vi "RPC Server-RT.vi"() -> ()   [LabVIEW 2020]
uses:
  <vilib>/Utility/error.llb/DialogType.ctl
  Lib/JSON-RPC/Classes/Server/Send Request (Sync).vi
  <vilib>/addons/analyzer/_analyzerutils.llb/VIAnUtil Check Type If ErrClust.vi
  Lib/JSON-RPC/Classes/Server/Add Response (Result).vi
  Lib/JSON-RPC/Classes/Server/Add Response (Internal Error).vi
  Lib/JSON-RPC/Classes/Server/Add Response (Method Not Found).vi
  Lib/JSON-RPC/Classes/Server/Add Response (Result from Request).vi
  Lib/JSON-RPC/Classes/Server/Add Response (Method Not Found from Request).vi
  Lib/JSON-RPC/Classes/Server/Add Response (Server Error from Request).vi
  Lib/JSON-RPC/Classes/Server/Add Response (Internal Error from Request).vi
  Lib/JSON-RPC/Classes/Server/JSONRPC Server.lvclass
  Controller/Controller.lvclass
  <vilib>/Utility/Data Type/NI_Data Type.lvlib
  <vilib>/NI_Real-Time Target Support.lvlib
  <vilib>/nisyscfg/nisyscfg.lvlib
panel:
  out "IP address":string
  out "header":string
  out "request":string
  out "response":string
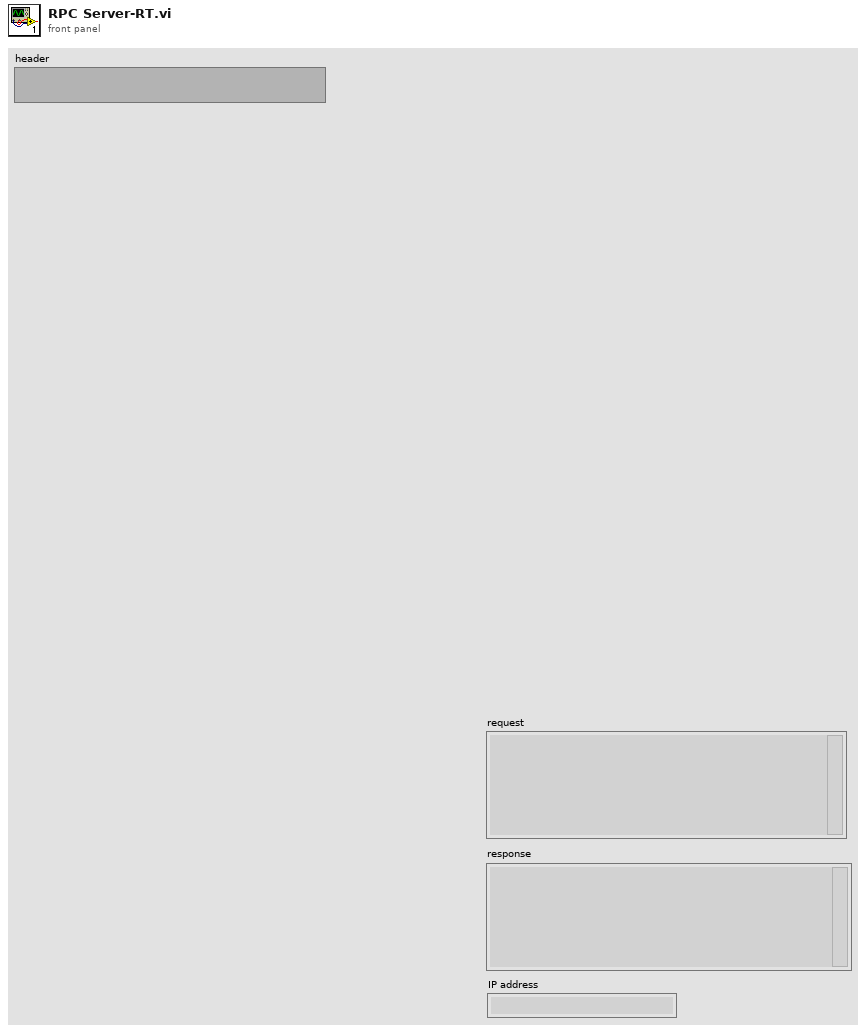
[diagram p1: front panel]
types:
  T1 = enum16{"Standard", "Buffered", "CRLF", "Immediate"}
  T2 = typedef "DialogType.ctl" = u16
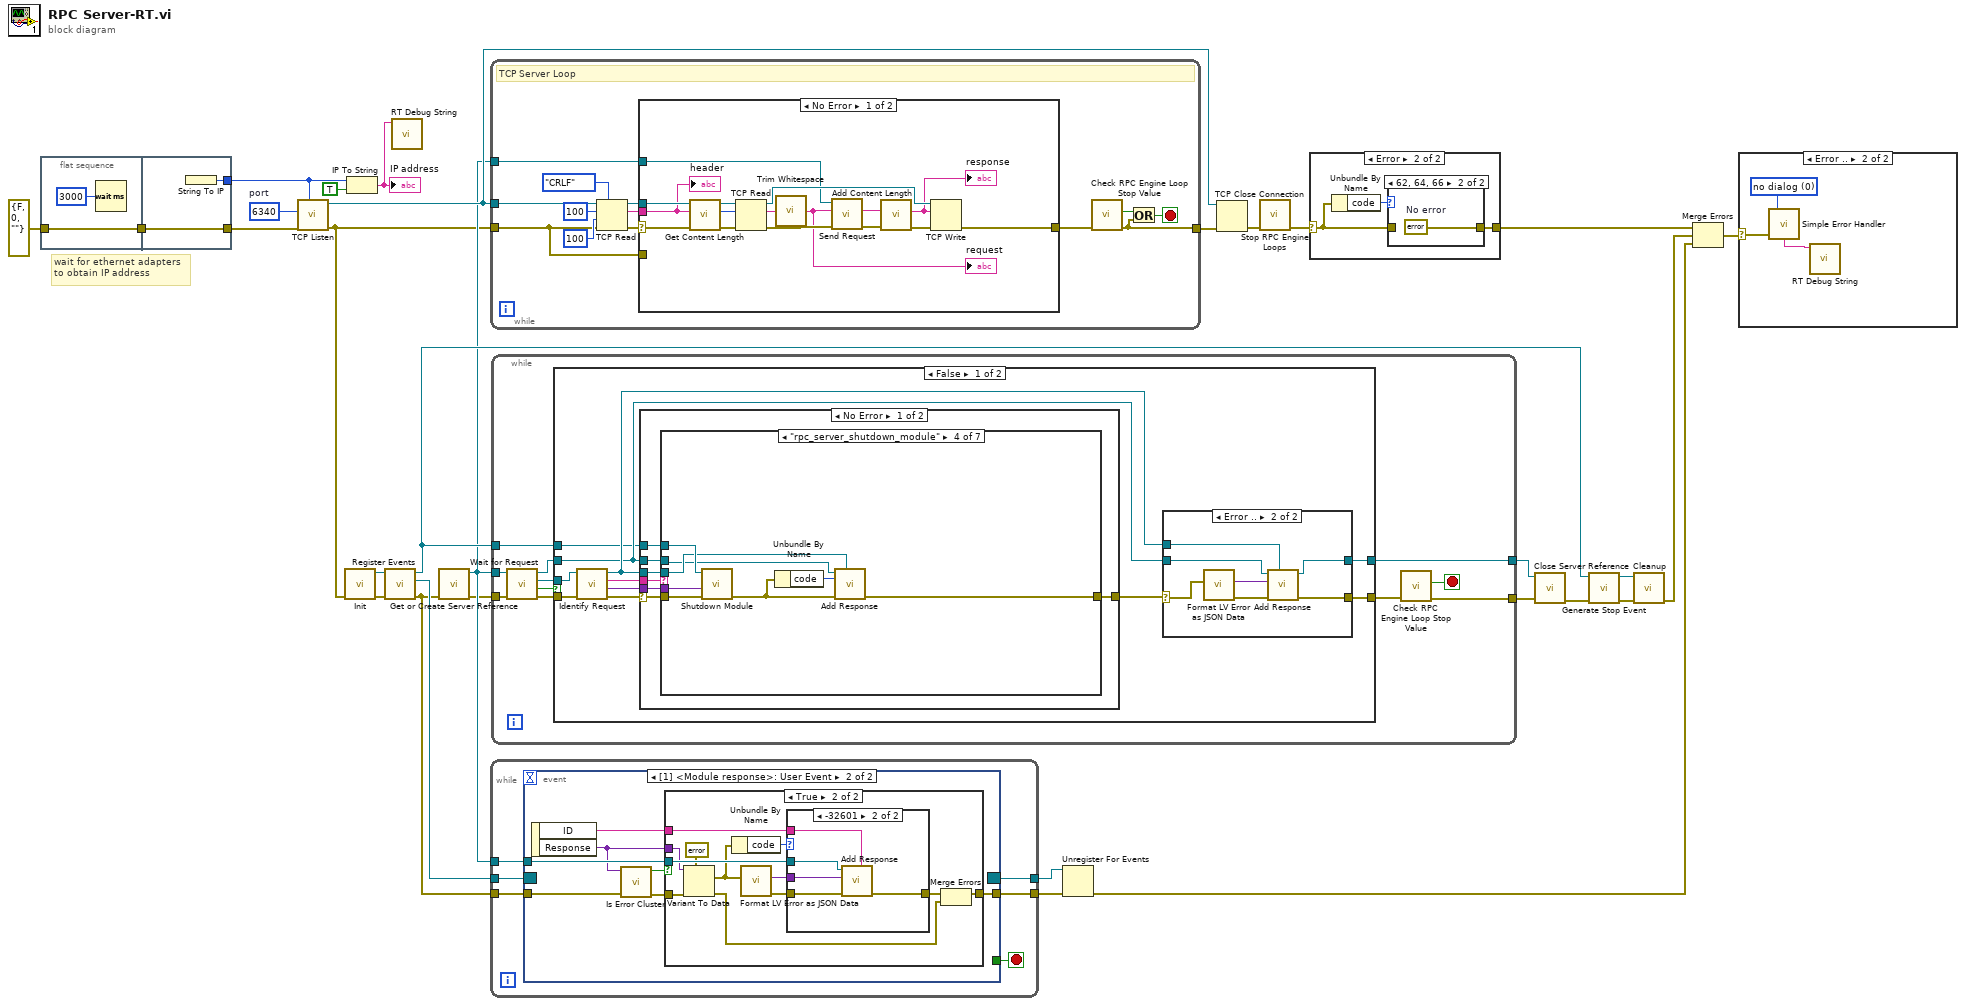
[diagram p0: block diagram]
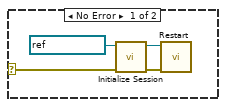
[diagram p2: hidden frame]
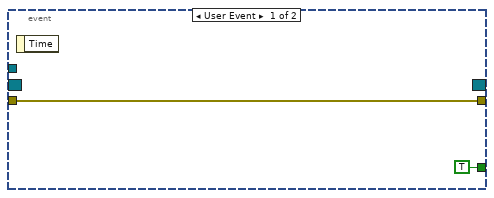
[diagram p3: hidden frame]
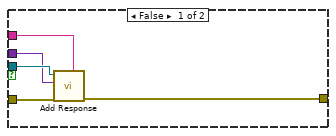
[diagram p4: hidden frame]
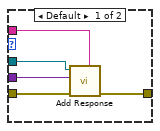
[diagram p5: hidden frame]
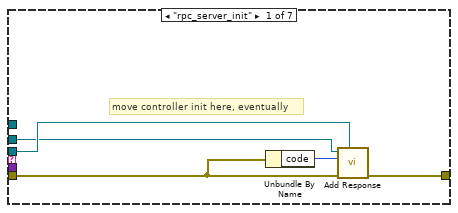
[diagram p7: hidden frame]
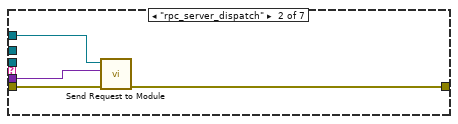
[diagram p8: hidden frame]
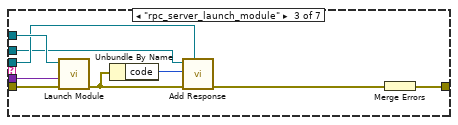
[diagram p9: hidden frame]
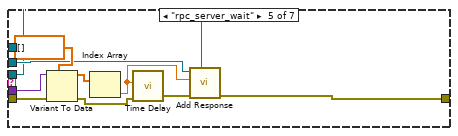
[diagram p10: hidden frame]
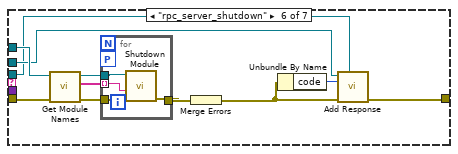
[diagram p11: hidden frame]
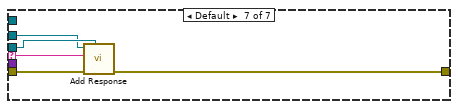
[diagram p12: hidden frame]
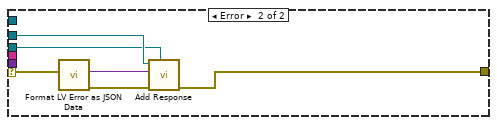
[diagram p13: hidden frame]
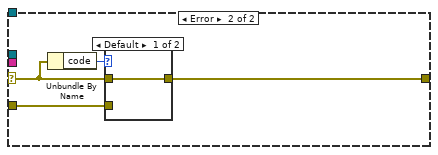
[diagram p17: hidden frame]
diagram:
  w29 = u16 6340  # port
  # "wait for ethernet adapters\nto obtain IP address"
  n1 = flat-sequence {
    tunnel: errorcluster {"status"=FALSE, "code"=0, "source"=""} ("error in (no error)") -> [w32]
    tunnel: [w32] -> w3
    tunnel: [w34] -> w6
    tunnel: w3 -> [w34]
    tunnel: [w33] -> w2
    frame #0 {
      n2 = Wait (ms)(milliseconds to wait=u32 3000) -> ()  [unwired: 1 out]
    }
    frame #1 {
      n3 = String To IP() -> (0:w33:u32)  [unwired: 1 in]
    }
  }
  n4 = call <vilib>:"TCP Listen.vi"("net address"=w2, "error in (no error)"=w6, "port"=w29) -> ("error out"=w4:errorcluster, "connection ID"=w26:refnum<k5>)  [unwired: 4 in, 3 out]
  n5 = call "Init.vi"("error in (no error)"=w4) -> ("error out"=w24:errorcluster, "Controller out"=w23:refnum<class "Controller.lvclass">)  [unwired: 9 in]
  n6 = IP To String(1:TRUE ("dot notation? (F)"), 2:w2) -> (0:w5:string)
  "IP address" <- w5
  n7 = call "Register Events.vi"("error in (no error)"=w24, "Controller in"=w23) -> ("error out"=w10:errorcluster, "Event Registration Refnum"=w22:refnum<event-registration>, "Controller out"=w15:refnum<class "Controller.lvclass">)  [unwired: 7 in]
  n8 = call <vilib>:"RT Debug String.vi"("String to write"=w5) -> ()  [unwired: 10 in, 1 out]
  n9 = call "Get or Create Server Reference.vi"("error in (no error)"=w10) -> ("error out"=w9:errorcluster, "Server Out"=w14:refnum<class "JSONRPC Server.lvclass">)  [unwired: 9 in]
  n10 = while {
    tunnel: [w35] -> w30
    tunnel: w26 -> [w41]
    tunnel: w4 -> [w42]
    tunnel: w14 -> [w39]
    stop <- w38 stop-if-true
    # "TCP Server Loop"
    n11 = TCP Read(connection ID=w41, bytes to read=100, error in (no error)=w42, 7:T1."CRLF" ("mode (standard)"), 9:100 ("timeout ms (25000)")) -> (connection ID out=w45:refnum<k5>, data out=w40:string, error out=w44:errorcluster)
    n12 = case shown="No Error" w44 {
      selector: w44 -> [w62 w65]
      tunnel: [w57 w64] -> w37
      tunnel: w42 -> [_ w63]
      tunnel: w45 -> [w60 _]
      tunnel: w40 -> [w59 _]
      tunnel: w39 -> [w51 _]
      frame No Error {
        n13 = call "Get Content Length.vi"("error in (no error)"=w62, "header"=w59) -> ("error out"=w61:errorcluster, "content length"=w58:i32)  [unwired: 8 in]
        n14 = TCP Read(connection ID=w60, bytes to read=w58, error in (no error)=w61) -> (connection ID out=w56:refnum<k5>, data out=w53:string, error out=w52:errorcluster)  [unwired: 2 out]
        n15 = call <vilib>:"Trim Whitespace.vi"("string"=w53) -> ("trimmed string"=w50:string)  [unwired: 1 in]
        "request" <- w50
        n16 = call-poly "Send Request.vi"("error in (no error)"=w52, "JSON Request String"=w50, "JSONRPC Server in"=w51) -> ("error out"=w48:errorcluster, "JSON Response String"=w49:string)  [unwired: 6 in, 1 out]
        n17 = call "Add Content Length.vi"("error in (no error)"=w48, "JSON Response String in"=w49) -> ("error out"=w55:errorcluster, "JSON Response String out"=w54:string)  [unwired: 8 in]
        "response" <- w54
        n18 = TCP Write(connection ID=w56, data in=w54, error in (no error)=w55) -> (error out=w57:errorcluster)  [unwired: 1 in, 2 out]
        "header" <- w59
      }
      frame Error {
        n19 = Unbundle By Name(w65) -> ("code"=w66:i32)
        n20 = case shown="Default" w66 {
          tunnel: w65 -> [w67 _]
          tunnel: w63 -> [_ w68]
          tunnel: [w67 w68] -> w64
          frame Default {
          }
          frame 56 {
          }
        }
      }
    }
    n21 = call "Check RPC Engine Loop Stop Value.vi"("error in (no error)"=w37) -> ("error out"=w35:errorcluster, "stopped?"=w36:bool)  [unwired: 9 in]
    n22 = Or(x=w36, y=w35) -> (x .or. y?=w38:bool)
  }
  n23 = while {
    tunnel: w22 -> [w74]
    tunnel: [w73] -> w21
    tunnel: w14 -> [w72]
    tunnel: w10 -> [w71]
    tunnel: [w70] -> w19
    stop <- w69 stop-if-true
    n24 = event shown="[1] <Module response>: User Event" {
      selector: w74 -> [_ _]
      dyn-events: [_ _] -> w73
      timeout: _ -> [_ _]
      tunnel: w72 -> [_ w81]
      tunnel: w71 -> [w76 w80]
      tunnel: [w76 w83] -> w70
      tunnel: [TRUE _] -> w69
      event User Event {
        n25 = event-data() -> ()  [unwired: 1 in, 1 out]
      }
      event User Event {
        n26 = event-data() -> ("ID"=w82:string, "Response"=w78:variant)  [unwired: 1 in]
        n27 = call <vilib>:"Is Error Cluster.vi"("error in (no error)"=w80, "variant"=w78) -> ("error out"=w79:errorcluster, "is error cluster?"=w77:bool)  [unwired: 8 in]
        n28 = case shown="True" w77 {
          tunnel: [w88 w98] -> w83
          tunnel: w82 -> [w87 w100]
          tunnel: w81 -> [w86 w99]
          tunnel: w79 -> [w85 w96]
          tunnel: w78 -> [w84 w94]
          frame False {
            n29 = call-poly "Add Response.vi"("id value"=w87, "error in (no error)"=w85, "JSON Value in"=w84, "Server in"=w86) -> ("error out"=w88:errorcluster)  [unwired: 5 in, 2 out]
          }
          frame True {
            n30 = Variant To Data(error in=w96, type=errorcluster {"status"=FALSE, "code"=0, "source"=""} ("data"), Variant=w94) -> (data=w91:errorcluster, error out=w95:errorcluster)
            n31 = Unbundle By Name(w91) -> ("code"=w92:i32)
            n32 = call "Format LV Error as JSON Data.vi"("error in"=w91) -> ("error out"=w89:errorcluster, "Error Value out"=w90:variant)  [unwired: 9 in]
            n33 = case shown="-32601" w92 {
              tunnel: w100 -> [w103 w108]
              tunnel: w99 -> [w105 w110]
              tunnel: [w104 w109] -> w97
              tunnel: w90 -> [w102 w107]
              tunnel: w89 -> [w101 w106]
              frame Default {
                n34 = call-poly "Add Response.vi"("id value"=w103, "error in (no error)"=w101, "JSON Value in"=w102, "Server in"=w105) -> ("error out"=w104:errorcluster)  [unwired: 5 in, 2 out]
              }
              frame -32601 {
                n35 = call-poly "Add Response.vi"("id value"=w108, "error in (no error)"=w106, "data"=w107, "Server in"=w110) -> ("error out"=w109:errorcluster)  [unwired: 5 in, 2 out]
              }
            }
            n36 = Merge Errors(w97, w95) -> (w98:errorcluster)
          }
        }
      }
    }
  }
  n37 = while {
    tunnel: w9 -> [w121]
    tunnel: w14 -> [w120]
    tunnel: [w112] -> w28
    tunnel: [w115] -> w27
    tunnel: w15 -> [w113]
    stop <- w111 stop-if-true
    n38 = call "Wait for Request.vi"("error in (no error)"=w121, "Server in"=w120) -> ("error out"=w119:errorcluster, "timed out?"=w116:bool, "Request"=w118:refnum<class "Request.lvclass">, "Server out"=w117:refnum<class "JSONRPC Server.lvclass">)  [unwired: 6 in]
    n39 = case shown="False" w116 {
      tunnel: w119 -> [w125 w212]
      tunnel: w118 -> [w132 _]
      tunnel: w117 -> [w123 w211]
      tunnel: [w128 w212] -> w114
      tunnel: [w127 w211] -> w115
      tunnel: w113 -> [w122 _]
      frame False {
        n40 = call "Identify Request.vi"("error in (no error)"=w125, "Request in"=w132) -> ("error out"=w126:errorcluster, "params"=w131:variant, "method"=w124:string, "Request out"=w129:refnum<class "Request.lvclass">)  [unwired: 5 in, 1 out]
        n41 = case shown="No Error" w126 {
          selector: w126 -> [w146 w210]
          tunnel: w131 -> [w143 _]
          tunnel: w123 -> [w148 w208]
          tunnel: w129 -> [w147 w207]
          tunnel: [w145 w205] -> w130
          tunnel: w124 -> [w144 _]
          tunnel: w122 -> [w142 _]
          frame No Error {
            n42 = case shown="\"rpc_server_shutdown_module\"" w144 {
              selector: w144 -> [_ _ _ _ _ _ w201]
              tunnel: w148 -> [w151 _ w160 w167 w178 w187 w202]
              tunnel: w147 -> [w152 _ w161 w168 w176 w185 w204]
              tunnel: w146 -> [w150 w157 w166 w174 w184 w190 w203]
              tunnel: [w153 w155 w165 w169 w175 w186 w200] -> w145
              tunnel: w143 -> [_ w154 w163 w172 w183 _ _]
              tunnel: w142 -> [_ w156 w164 w173 _ w191 _]
              frame "rpc_server_init" {
                # "move controller init here, eventually"
                n43 = Unbundle By Name(w150) -> ("code"=w149:i32)
                n44 = call-poly "Add Response.vi"("Request"=w152, "error in (no error)"=w150, "JSON Value in"=w149, "Server in"=w151) -> ("error out"=w153:errorcluster)  [unwired: 5 in, 2 out]
              }
              frame "rpc_server_dispatch" {
                n45 = call "Send Request to Module.vi"("error in (no error)"=w157, "Request"=w154, "Controller in"=w156) -> ("error out"=w155:errorcluster)  [unwired: 6 in, 2 out]
              }
              frame "rpc_server_launch_module" {
                n46 = call "Launch Module.vi"("error in (no error)"=w166, "params"=w163, "Controller in"=w164) -> ("error out"=w159:errorcluster)  [unwired: 7 in, 1 out]
                n47 = Unbundle By Name(w159) -> ("code"=w158:i32)
                n48 = call-poly "Add Response.vi"("Request"=w161, "error in (no error)"=w159, "JSON Value in"=w158, "Server in"=w160) -> ("error out"=w162:errorcluster)  [unwired: 5 in, 2 out]
                n49 = Merge Errors(w162) -> (w165:errorcluster)
              }
              frame "rpc_server_shutdown_module" {
                n50 = call "Shutdown Module.vi"("error in (no error)"=w174, "params"=w172, "Controller in"=w173) -> ("error out"=w170:errorcluster)  [unwired: 7 in, 1 out]
                n51 = Unbundle By Name(w170) -> ("code"=w171:i32)
                n52 = call-poly "Add Response.vi"("Request"=w168, "error in (no error)"=w170, "JSON Value in"=w171, "Server in"=w167) -> ("error out"=w169:errorcluster)  [unwired: 5 in, 2 out]
              }
              frame "rpc_server_wait" {
                n53 = Variant To Data(error in=w184, type=dbl[] [], Variant=w183) -> (data=w181:dbl[], error out=w180:errorcluster)
                n54 = Index Array(array=w181) -> (element=w177:dbl)  [unwired: 1 in]
                n55 = call "Time Delay"("error in (no error)"=w180, "Delay Time (s)"=w177) -> ("error out"=w179:errorcluster)  [unwired: 9 in]
                n56 = call-poly "Add Response.vi"("Request"=w176, "error in (no error)"=w179, "JSON Value in"=w177, "Server in"=w178) -> ("error out"=w175:errorcluster)  [unwired: 5 in, 2 out]
              }
              frame "rpc_server_shutdown" {
                n57 = call "Get Module Names.vi"("error in (no error)"=w190, "Controller in"=w191) -> ("error out"=w194:errorcluster, "Names"=w195:string[], "Controller out"=w192:refnum<class "Controller.lvclass">)  [unwired: 7 in]
                n58 = for {
                  tunnel: w192 -> [w199]
                  tunnel: w195 -> [w196] mode=indexing
                  tunnel: w194 -> [w198]
                  tunnel: [w197] -> _ mode=indexing
                  tunnel: [w197] -> w193
                  workers-P: _ -> [_]
                  n59 = call "Shutdown Module.vi"("error in (no error)"=w198, "params"=w196, "Controller in"=w199) -> ("error out"=w197:errorcluster)  [unwired: 7 in, 1 out]
                }
                n60 = Merge Errors(w193) -> (w189:errorcluster)
                n61 = Unbundle By Name(w189) -> ("code"=w188:i32)
                n62 = call-poly "Add Response.vi"("Request"=w185, "error in (no error)"=w189, "JSON Value in"=w188, "Server in"=w187) -> ("error out"=w186:errorcluster)  [unwired: 5 in, 2 out]
              }
              frame Default {
                n63 = call-poly "Add Response.vi"("Request"=w204, "error in (no error)"=w203, "data"=w201, "Server in"=w202) -> ("error out"=w200:errorcluster)  [unwired: 5 in, 2 out]
              }
            }
          }
          frame Error {
            n64 = call "Format LV Error as JSON Data.vi"("error in"=w210) -> ("error out"=w209:errorcluster, "Error Value out"=w206:variant)  [unwired: 9 in]
            n65 = call-poly "Add Response.vi"("Request"=w207, "error in (no error)"=w209, "data"=w206, "Server in"=w208) -> ("error out"=w205:errorcluster)  [unwired: 5 in, 2 out]
          }
        }
        n66 = case shown="Error .." w130 {
          selector: w130 -> [w134 w139]
          tunnel: [w134 w138] -> w128
          tunnel: w123 -> [w133 w136]
          tunnel: [w133 w137] -> w127
          tunnel: w129 -> [_ w135]
          frame No Error {
          }
          frame Error {
            n67 = call "Format LV Error as JSON Data.vi"("error in"=w139) -> ("error out"=w141:errorcluster, "Error Value out"=w140:variant)  [unwired: 9 in]
            n68 = call-poly "Add Response.vi"("Request"=w135, "error in (no error)"=w141, "data"=w140, "Server in"=w136) -> ("error out"=w138:errorcluster, "Server out"=w137:refnum<class "JSONRPC Server.lvclass">)  [unwired: 5 in, 1 out]
          }
        }
      }
      frame True {
      }
    }
    n69 = call "Check RPC Engine Loop Stop Value.vi"("error in (no error)"=w114) -> ("error out"=w112:errorcluster, "stopped?"=w111:bool)  [unwired: 9 in]
  }
  n70 = Unregister For Events(event registration refnum=w21, error in=w19) -> (error out=w20:errorcluster)
  n71 = TCP Close Connection(connection ID=w26, error in (no error)=w30) -> (error out=w13:errorcluster)  [unwired: 2 out]
  n72 = call "Stop RPC Engine Loops.vi"("error in (no error)"=w13) -> ("error out"=w12:errorcluster)  [unwired: 10 in]
  n73 = case shown="Error" w12 {
    selector: w12 -> [w213 w215]
    tunnel: [w213 w214] -> w11
    frame No Error {
    }
    frame Error {
      n74 = Unbundle By Name(w215) -> ("code"=w216:i32)
      n75 = case shown="62, 64, 66" w216 {
        tunnel: w215 -> [w217 _]
        tunnel: [w217 w218] -> w214
        frame Default {
        }
        frame 62, 64, 66 {
          w218 = errorcluster {"status"=FALSE, "code"=0, "source"=""}  # No error
        }
      }
    }
  }
  n76 = call "Close Server Reference.vi"("error in (no error)"=w28, "Server in"=w27) -> ("error out"=w16:errorcluster)  [unwired: 9 in]
  n77 = call "Generate Stop Event.vi"("error in (no error)"=w16, "Controller in"=w15) -> ("error out"=w18:errorcluster, "Controller out"=w17:refnum<class "Controller.lvclass">)  [unwired: 8 in]
  n78 = call "Cleanup.vi"("error in (no error)"=w18, "Controller in"=w17) -> ("error out"=w25:errorcluster)  [unwired: 9 in]
  n79 = Merge Errors(w11, w25, w20) -> (w1:errorcluster)
  n80 = case shown="Error .." w1 {
    selector: w1 -> [w220 w225]
    frame No Error {
      n81 = call <vilib>:"Initialize Session.vi"("error in (no error)"=w220, "Target (localhost)"=refnum<k21> "localhost") -> ("error out"=w221:errorcluster, "Session out"=w222:refnum<k21>)  [unwired: 8 in]
      n82 = call <vilib>:"Restart.vi"("error in (no error)"=w221, "Session in"=w222) -> ()  [unwired: 7 in, 3 out]
    }
    frame Error {
      w224 = T2 0 items=["no dialog", "OK message", "continue or stop message", "OK message + warnings", "continue/stop + warnings"] ("type of dialog (OK msg:1)")
      n83 = call <vilib>:"Simple Error Handler.vi"("type of dialog (OK msg:1)"=w224, "error in (no error)"=w225) -> ("message"=w223:string)  [unwired: 3 in, 4 out]
      n84 = call <vilib>:"RT Debug String.vi"("String to write"=w223) -> ()  [unwired: 10 in, 1 out]
    }
  }
